vi "thermistor_read_Joe_2.vi"(0 "Arduino Resource":T1={"VISA resource"="COM11", "Board Type"=enum."Uno", "Connection Type"=enum."USB / Serial", "Bytes Per Packet (15)"=15}, 1 "Units (C)":enum16{"Celsius", "Fahrenheit", "Kelvin"}(ring), 5 "Thermistor AI Pin (0)":u8, 7 "Paired Resistance (10K Ohms)":dbl=10000.0, 9 "Vcc (5 v)":dbl=5.0, 11 "error in":errorcluster) -> (4 "Arduino Resource":T1={"VISA resource"="COM11", "Board Type"=enum."Uno", "Connection Type"=enum."USB / Serial", "Bytes Per Packet (15)"=15}, 8 "Temperature":dbl, 15 "error out":errorcluster)   [LabVIEW 2011]
doc: "Read the temperature from a thermistor. Thermistor must be used in a voltage divider with a paired resistance. The paired resistance is user selectable however a value of 10K Ohms is recommended.\n\nThe constant for the Steinhart-Hart are changed to match the values given for our NTC."
uses:
  <vilib>/LabVIEW Interface for Arduino/Type Defs/Arduino Resource.ctl
  <vilib>/LabVIEW Interface for Arduino/Type Defs/Board Type.ctl
  <vilib>/express/express arith-compare/Formula/XNode/ExpressFormulaBlockNode.xnode
  <vilib>/LabVIEW Interface for Arduino/LabVIEW Interface for Arduino.lvlib
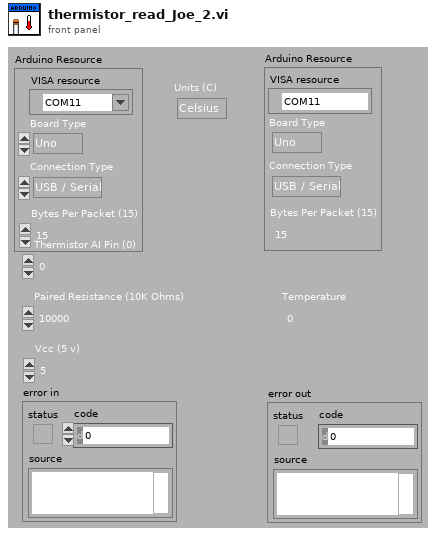
[diagram p1: front panel]
types:
  T1 = typedef "LabVIEW Interface for Arduino.lvlib/Arduino Resource.ctl" = cluster{"VISA resource":refnum<visa-resource-name>, "Board Type":T2, "Connection Type":enum8{"USB / Serial"}, "Bytes Per Packet (15)":u8}
  T2 = typedef "LabVIEW Interface for Arduino.lvlib/Board Type.ctl" = enum16{"Uno", "Dimuelanove w/Atmega 328", "Mega 2560"}
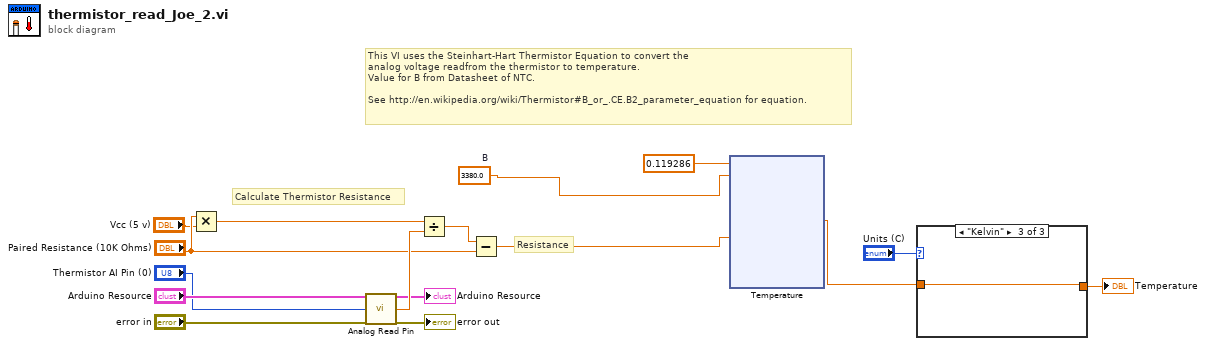
[diagram p0: block diagram]
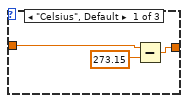
[diagram p2: hidden frame]
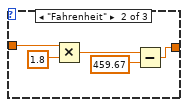
[diagram p3: hidden frame]
diagram:
  w2 = 3380.0  # B
  # "Resistance"
  # "This VI uses the Steinhart-Hart Thermistor Equation to convert the \nanalog voltage readfrom the thermistor to temperature.\nValue for B from Datasheet of NTC.\n\nSee http://en.wikipedia.org/wiki/Thermistor#B_or_.CE.B2_parameter_equation for equation."
  # "Calculate Thermistor Resistance"
  n1 = Multiply(x="Paired Resistance (10K Ohms)", y="Vcc (5 v)") -> (x*y=w16:dbl)
  n2 = call <vilib>:"Analog Read Pin.vi"("Arduino Resource"="Arduino Resource", "Analog Input Pin (0)"="Thermistor AI Pin (0)", "error in"="error in") -> ("Arduino Resource"=→"Arduino Resource":T1, "Voltage"=w15:dbl, "error out"=→"error out":errorcluster)  [unwired: 10 in]
  n3 = Divide(x=w16, y=w15) -> (x/y=w14:dbl)
  n4 = Subtract(x=w14, y="Paired Resistance (10K Ohms)") -> (x-y=w4:dbl)
  n5 = xnode ("Temperature")("R"=w4, "r_inf"=0.119286, "B"=w2) -> ("Result"=w3:dbl)  [unwired: 1 in, 1 out]
  n6 = case shown="\"Kelvin\"" "Units (C)" {
    tunnel: [w18 w21 w25] -> w8
    tunnel: w3 -> [w17 w20 w25]
    frame "Celsius", Default {
      n7 = Subtract(x=w17, y=273.15) -> (x-y=w18:dbl)
    }
    frame "Fahrenheit" {
      n8 = Multiply(x=w20, y=1.8) -> (x*y=w23:dbl)
      n9 = Subtract(x=w23, y=459.67) -> (x-y=w21:dbl)
    }
    frame "Kelvin" {
    }
  }
  "Temperature" <- w8
